vi "RPi_I2C_BME280_Calibration_Read.vi"(0 "LINX Resource":T2, 1 "I2C Channel (0)":u8, 2 "I2C Slave Address (0)":u8, 11 "error in (no error)":errorcluster) -> (4 "LINX Resource out":T2, 6 "Calibration Coefficients":T1, 15 "error out":errorcluster)   [LabVIEW 2020]
doc: "Reads the BME280 Calibration Coefficients using the I2C protocol.\n\nFirst reads the Calibration Registers, than converts the Registers to Raw Calibration Coefficients.\n\nMIT License\nCopyright (c) 2021 Asper"
uses:
  <vilib>/MakerHub/LINX/Private/Type Defs/LINX Ref.ctl
  <vilib>/MakerHub/LINX/Private/Type Defs/Platform.ctl
  <vilib>/MakerHub/LINX/Private/Type Defs/Interface.ctl
  <vilib>/MakerHub/LINX/Private/Device/Type Defs/LINX Device Config.ctl
  <vilib>/MakerHub/LINX/Private/Device/Type Defs/TCP Config.ctl
  <vilib>/MakerHub/LINX/Private/Device/Type Defs/Channels.ctl
  Type_Def/BME280_Calibration_Coefficients.ctl
  <vilib>/MakerHub/LINX/LMH-LINX.lvlib
  <vilib>/MakerHub/LINX/Private/Device/Device.lvlib
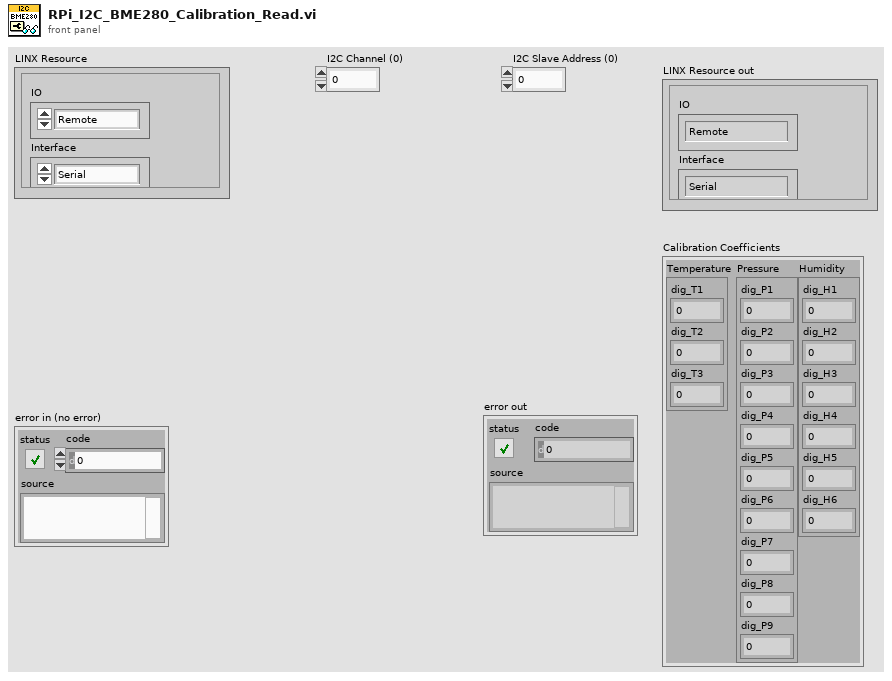
[diagram p1: front panel]
types:
  T1 = typedef "BME280_Calibration_Coefficients.ctl" = cluster{"Temperature":cluster{"dig_T1":u16, "dig_T2":i16, "dig_T3":i16}, "Pressure":cluster{"dig_P1":u16, "dig_P2":i16, "dig_P3":i16, "dig_P4":i16, "dig_P5":i16, "dig_P6":i16, "dig_P7":i16, "dig_P8":i16, "dig_P9":i16}, "Humidity":cluster{"dig_H1":u8, "dig_H2":i16, "dig_H3":u8, "dig_H4":i16, "dig_H5":i16, "dig_H6":i8}}
  T2 = typedef "LMH-LINX.lvlib/LINX Ref.ctl" = cluster{"IO":T3, "Interface":T4, "LINX Device Config":T5}
  T3 = typedef "LMH-LINX.lvlib/Platform.ctl" = enum16{"Remote", "Local"}
  T4 = typedef "LMH-LINX.lvlib/Interface.ctl" = enum16{"Serial", "TCP"}
  T5 = typedef "LMH-LINX.lvlib/Device.lvlib/LINX Device Config.ctl" = cluster{"Interface":T4, "COM Port":refnum<visa-resource-name>, "TCP Configuration":T6, "Device Family":u8, "Device ID":u8, "Device Name":string, "TCP Ref":refnum<k5>, "Channels":T7}
  T6 = typedef "LMH-LINX.lvlib/Device.lvlib/TCP Config.ctl" = cluster{"IP Address":string, "Port":u16}
  T7 = typedef "LMH-LINX.lvlib/Channels.ctl" = cluster{"DI":u8[], "DO":u8[], "AI":u8[], "AO":u8[], "PWM":u8[], "QE":u8[], "UART":u8[], "I2C 2":u8[], "SPI":u8[], "CAN":u8[], "Servo":u8[], "AI Ref (V)":dbl, "AI Resolution (Bits)":u8, "AO Ref (V)":dbl, "AO Resolution (Bits)":u8}
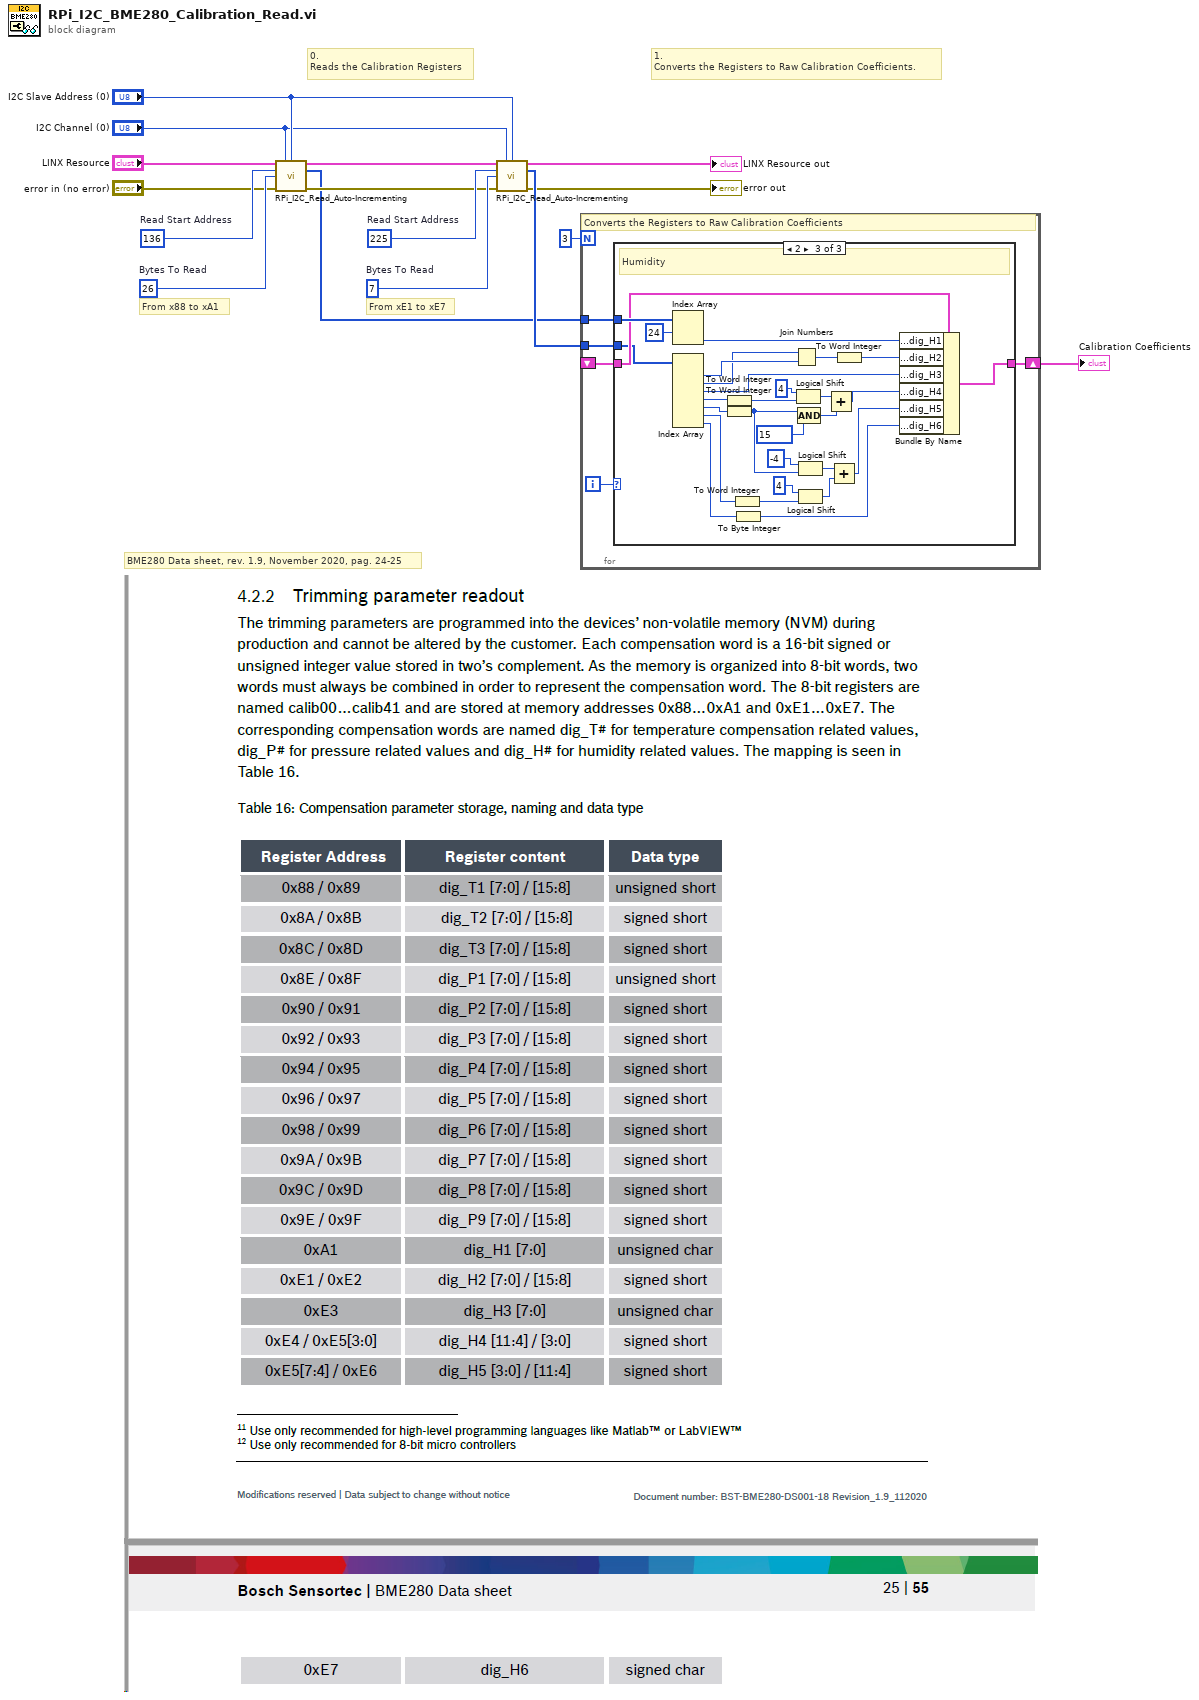
[diagram p0: block diagram]
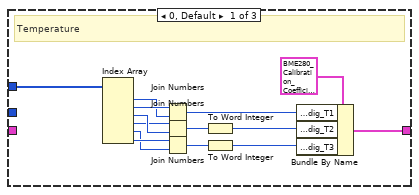
[diagram p2: hidden frame]
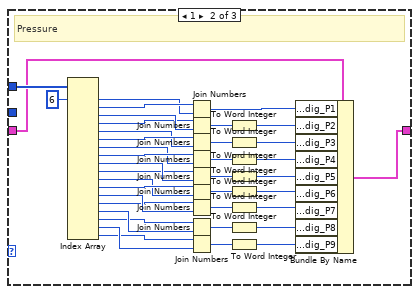
[diagram p3: hidden frame]
diagram:
  w15 = u8 7  # Bytes To Read
  w14 = u8 225  # Read Start Address
  w5 = u8 26  # Bytes To Read
  w6 = u8 136  # Read Start Address
  # "1.\nConverts the Registers to Raw Calibration Coefficients."
  # "0.\nReads the Calibration Registers"
  # "From xE1 to xE7"
  # "From x88 to xA1"
  # "BME280 Data sheet, rev. 1.9, November 2020, pag. 24-25"
  n1 = call "RPi_I2C_Read_Auto-Incrementing.vi"("LINX Resource in"="LINX Resource", "I2C Channel (0)"="I2C Channel (0)", "I2C Slave Address (0)"="I2C Slave Address (0)", "Start Register Address"=w6, "Number of Bytes To Read"=w5, "error in (no error)"="error in (no error)") -> ("LINX Resource out"=w8:T2, "Registers (Bytes)"=w7:u8[], "error out"=w9:errorcluster)  [unwired: 7 in]
  n2 = call "RPi_I2C_Read_Auto-Incrementing.vi"("LINX Resource in"=w8, "I2C Channel (0)"="I2C Channel (0)", "I2C Slave Address (0)"="I2C Slave Address (0)", "Start Register Address"=w14, "Number of Bytes To Read"=w15, "error in (no error)"=w9) -> ("LINX Resource out"=→"LINX Resource out":T2, "Registers (Bytes)"=w16:u8[], "error out"=→"error out":errorcluster)  [unwired: 7 in]
  n3 = for {
    N: 3 -> [_]
    tunnel: w7 -> [w21]
    shift-right: [w20] -> w2
    shift-left: _ -> [w19]
    tunnel: w16 -> [w17]
    i -> [w18]
    # "Converts the Registers to Raw Calibration Coefficients"
    n4 = case shown="2" w18 {
      tunnel: w21 -> [w33 w72 w103]
      tunnel: [w23 w62 w100] -> w20
      tunnel: w19 -> [_ w61 w99]
      tunnel: w17 -> [_ _ w96]
      frame 0, Default {
        # "Temperature"
        n5 = Index Array(array=w33) -> (element #1=w34:u8, element #2=w35:u8, element #3=w32:u8, element #4=w31:u8, element #5=w29:u8, element #6=w30:u8)  [unwired: 6 in]
        n6 = Join Numbers(hi=w35, lo=w34) -> ((hi.lo)=w26:u16)
        n7 = Join Numbers(hi=w31, lo=w32) -> ((hi.lo)=w28:u16)
        n8 = Join Numbers(hi=w30, lo=w29) -> ((hi.lo)=w27:u16)
        n9 = To Word Integer(number=w28) -> (16bit integer=w25:i16)
        n10 = To Word Integer(number=w27) -> (16bit integer=w24:i16)
        n11 = Bundle By Name(cluster=T1 {"Temperature"={"dig_T1"=0, "dig_T2"=0, "dig_T3"=0}, "Pressure"={"dig_P1"=0, "dig_P2"=0, "dig_P3"=0, "dig_P4"=0, "dig_P5"=0, "dig_P6"=0, "dig_P7"=0, "dig_P8"=0, "dig_P9"=0}, "Humidity"={"dig_H1"=0, "dig_H2"=0, "dig_H3"=0, "dig_H4"=0, "dig_H5"=0, "dig_H6"=0}} ("Calibration Coefficients"), "Temperature.dig_T1"=w26, "Temperature.dig_T2"=w25, "Temperature.dig_T3"=w24) -> (w23:T1)
      }
      frame 1 {
        # "Pressure"
        n12 = Index Array(array=w72, index #1=6 ("index")) -> (element #1=w73:u8, element #2=w74:u8, element #3=w71:u8, element #4=w70:u8, element #5=w68:u8, element #6=w69:u8, element #7=w47:u8, element #8=w48:u8, element #9=w46:u8, element #10=w45:u8, element #11=w43:u8, element #12=w44:u8, element #13=w42:u8, element #14=w41:u8, element #15=w40:u8, element #16=w39:u8, element #17=w38:u8, element #18=w37:u8)  [unwired: 17 in]
        n13 = Join Numbers(hi=w74, lo=w73) -> ((hi.lo)=w65:u16)
        n14 = Join Numbers(hi=w70, lo=w71) -> ((hi.lo)=w67:u16)
        n15 = Join Numbers(hi=w69, lo=w68) -> ((hi.lo)=w66:u16)
        n16 = Join Numbers(hi=w48, lo=w47) -> ((hi.lo)=w58:u16)
        n17 = Join Numbers(hi=w45, lo=w46) -> ((hi.lo)=w60:u16)
        n18 = Join Numbers(hi=w44, lo=w43) -> ((hi.lo)=w56:u16)
        n19 = Join Numbers(hi=w41, lo=w42) -> ((hi.lo)=w59:u16)
        n20 = Join Numbers(hi=w39, lo=w40) -> ((hi.lo)=w55:u16)
        n21 = Join Numbers(hi=w37, lo=w38) -> ((hi.lo)=w57:u16)
        n22 = To Word Integer(number=w67) -> (16bit integer=w64:i16)
        n23 = To Word Integer(number=w66) -> (16bit integer=w63:i16)
        n24 = To Word Integer(number=w58) -> (16bit integer=w54:i16)
        n25 = To Word Integer(number=w60) -> (16bit integer=w53:i16)
        n26 = To Word Integer(number=w56) -> (16bit integer=w52:i16)
        n27 = To Word Integer(number=w59) -> (16bit integer=w51:i16)
        n28 = To Word Integer(number=w55) -> (16bit integer=w50:i16)
        n29 = To Word Integer(number=w57) -> (16bit integer=w49:i16)
        n30 = Bundle By Name(cluster=w61, "Pressure.dig_P1"=w65, "Pressure.dig_P2"=w64, "Pressure.dig_P3"=w63, "Pressure.dig_P4"=w54, "Pressure.dig_P5"=w53, "Pressure.dig_P6"=w52, "Pressure.dig_P7"=w51, "Pressure.dig_P8"=w50, "Pressure.dig_P9"=w49) -> (w62:T1)
      }
      frame 2 {
        # "Humidity"
        n31 = Index Array(array=w103, index #1=24 ("index")) -> (element #2=w97:u8)  [unwired: 1 in, 1 out]
        n32 = Index Array(array=w96) -> (element #1=w95:u8, element #2=w94:u8, element #3=w93:u8, element #4=w92:u8, element #5=w88:u8, element #6=w80:u8, element #7=w76:u8)  [unwired: 7 in]
        n33 = To Word Integer(number=w92) -> (16bit integer=w91:i16)
        n34 = To Word Integer(number=w88) -> (16bit integer=w84:i16)
        n35 = To Word Integer(number=w80) -> (16bit integer=w82:i16)
        n36 = To Byte Integer(number=w76) -> (8bit integer=w75:i8)
        n37 = Join Numbers(hi=w94, lo=w95) -> ((hi.lo)=w102:u16)
        n38 = Logical Shift(y=i16 4, x=w91) -> (x << y=w89:i16)
        n39 = Logical Shift(y=i16 -4, x=w84) -> (x << y=w79:i16)
        n40 = Logical Shift(y=i16 4, x=w82) -> (x << y=w78:i16)
        n41 = Compound Arithmetic op=AND ("複合演算")(w84, i16 15 ("値")) -> (w87:i16)
        n42 = Add(x=w89, y=w87) -> (x+y=w86:i16)
        n43 = Add(x=w79, y=w78) -> (x+y=w77:i16)
        n44 = To Word Integer(number=w102) -> (16bit integer=w101:i16)
        n45 = Bundle By Name(cluster=w99, "Humidity.dig_H1"=w97, "Humidity.dig_H2"=w101, "Humidity.dig_H3"=w93, "Humidity.dig_H4"=w86, "Humidity.dig_H5"=w77, "Humidity.dig_H6"=w75) -> (w100:T1)
      }
    }
  }
  "Calibration Coefficients" <- w2
